vi "sudoku_solver_csv.vi"() -> ()   [LabVIEW 2019]
uses:
  <vilib>/Utility/error.llb/DialogType.ctl
  <vilib>/Utility/file.llb/Write Delimited Spreadsheet (DBL).vi
  <vilib>/Utility/file.llb/Read Delimited Spreadsheet (DBL).vi
panel:
  in  "Input string":string
  out "Array OUT":dbl[][](array[numeric])
  in  "Array IN":dbl[][](array[numeric])
  out "standard error":string
  out "standard output":string="19.0\r\n"
  # "solve = solve puzzle"
  # "clear = clear the output"
  # "Sudoku solves when Input is : solve"
  # "Clear the output when the output is: clear"
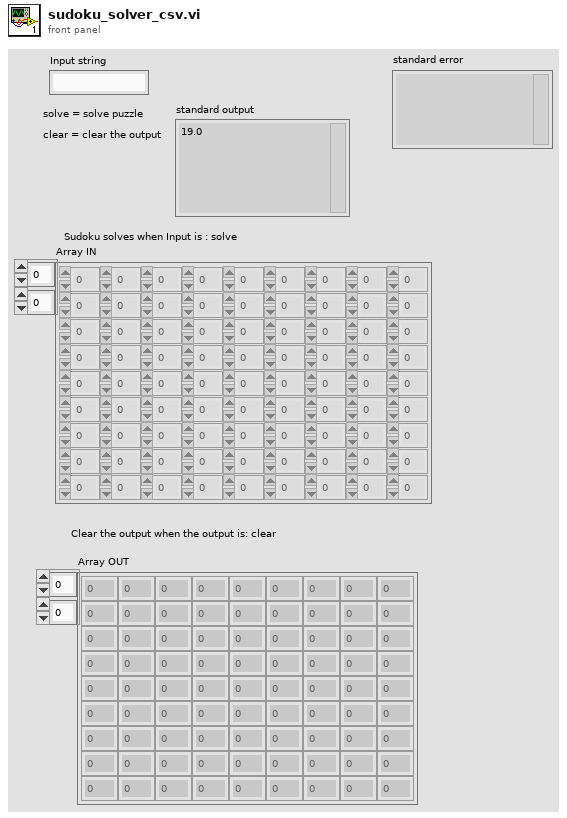
[diagram p1: front panel]
types:
  T1 = typedef "DialogType.ctl" = u16
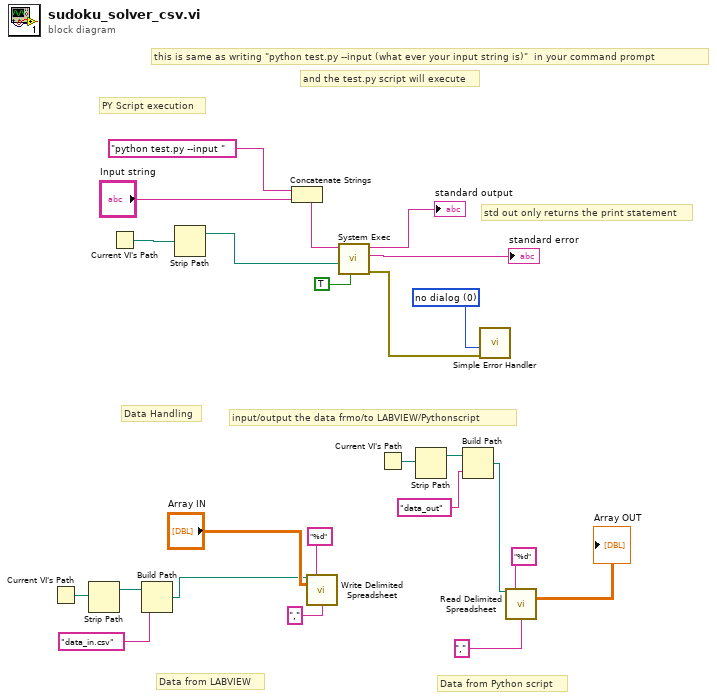
[diagram p0: block diagram]
diagram:
  w16 = T1 0 items=["no dialog", "OK message", "continue or stop message", "OK message + warnings", "continue/stop + warnings"] ("type of dialog (OK msg:1)")
  # "and the test.py script will execute"
  # "input/output the data frmo/to LABVIEW/Pythonscript"
  # "std out only returns the print statement"
  # "this is same as writing \"python test.py --input (what ever your input string is)\"  in your command prompt"
  # "Data from Python script"
  # "Data from LABVIEW"
  # "PY Script execution"
  # "Data Handling"
  n1 = Current VI's Path() -> (path=w9:path)
  n2 = Strip Path(path=w9) -> (stripped path=w8:path)  [unwired: 1 out]
  n3 = Current VI's Path() -> (path=w24:path)
  n4 = Build Path(base path=w8, name or relative path="data_in.csv") -> (appended path=w6:path)
  n5 = Strip Path(path=w24) -> (stripped path=w23:path)  [unwired: 1 out]
  n6 = Concatenate Strings("python test.py --input ", "Input string") -> (w21:string)
  n7 = call-poly <vilib>:"Write Delimited Spreadsheet.vi"("file path (dialog if empty)"=w6, "format (%.3f)"="%d", "2D data"="Array IN", "delimiter (\\t)"="," ("delimiter (\\t)")) -> ()  [unwired: 10 in, 2 out]
  n8 = call <vilib>:"System Exec.vi"("run minimized? (F)"=TRUE, "working directory"=w23, "command line"=w21) -> ("error out"=w17:errorcluster, "standard error"=→"standard error":string, "standard output"=→"standard output":string)  [unwired: 5 in, 1 out]
  n9 = Current VI's Path() -> (path=w5:path)
  n10 = Strip Path(path=w5) -> (stripped path=w4:path)  [unwired: 1 out]
  n11 = Build Path(base path=w4, name or relative path="data_out") -> (appended path=w2:path)
  n12 = call <vilib>:"Simple Error Handler.vi"("type of dialog (OK msg:1)"=w16, "error in (no error)"=w17) -> ()  [unwired: 3 in, 5 out]
  n13 = call-poly <vilib>:"Read Delimited Spreadsheet.vi"("file path (dialog if empty)"=w2, "format (%.3f)"="%d", "delimiter (\\t)"="," ("delimiter (\\t)")) -> ("all rows"=→"Array OUT":dbl[][])  [unwired: 7 in, 5 out]
